vi "LedDisplay.vi"(10 "字符串":string, 11 "L 2":refnum<vi>) -> (3 "引用输出":refnum<vi>)   [LabVIEW 2018]
panel:
  out "L 1":bool
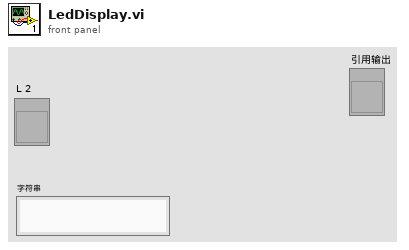
[diagram p1: front panel]
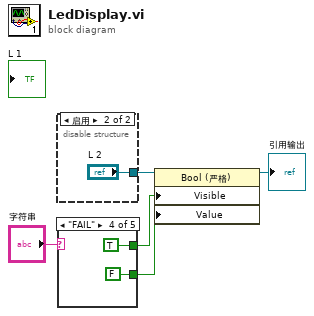
[diagram p0: block diagram]
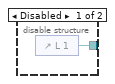
[diagram p2: hidden frame]
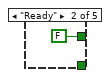
[diagram p4: hidden frame]
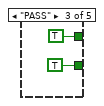
[diagram p5: hidden frame]
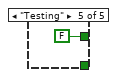
[diagram p6: hidden frame]
diagram:
  n1 = disable-structure shown="启用" {
    disable-tunnel: [w6 "L 2"] -> w5
    frame Disabled {
      n2 = control-ref of="L 1"() -> (w6:refnum<vi>)
    }
    frame Enabled {
    }
  }
  n3 = case shown="\"FAIL\"" "字符串" {
    tunnel: [_ FALSE TRUE TRUE FALSE] -> w3
    tunnel: [_ _ TRUE FALSE _] -> w1
    frame "假", Default {
    }
    frame "Ready" {
    }
    frame "PASS" {
    }
    frame "FAIL" {
    }
    frame "Testing" {
    }
  }
  n4 = property on="属性节点" class="Bool (严格)"(reference=w5, "Visible"=w3, "Value"=w1) -> (reference out=→"引用输出":refnum<vi>)  [unwired: 1 in, 1 out]
